vi "DebugView.vi"(10 "Compiled.Settings.ctl":T1, 11 "appended array":T8(array[cluster]) {"VS Refs" format="%.0x"}) -> ()   [LabVIEW 2019]
uses:
  <vilib>/NI VeriStand/Custom Device API/Custom Device Item Ref.ctl
  Shared/Compiled.Settings.ctl
  Shared/main_page_config.ctl
  Shared/object_managament_config.ctl
  Shared/interaction_parameter_configuration.ctl
  Shared/object_attribute_configuration.ctl
  Shared/object_status_info.ctl
  <vilib>/NI VeriStand/Custom Device API/Custom Device API.lvlib
  Shared/HLA Custom Device Shared.lvlib
panel:
  out "Compiled.Settings.ctl view":T1
  out "appended array view":T8(array[cluster]) {"VS Refs" format="%.0x"}
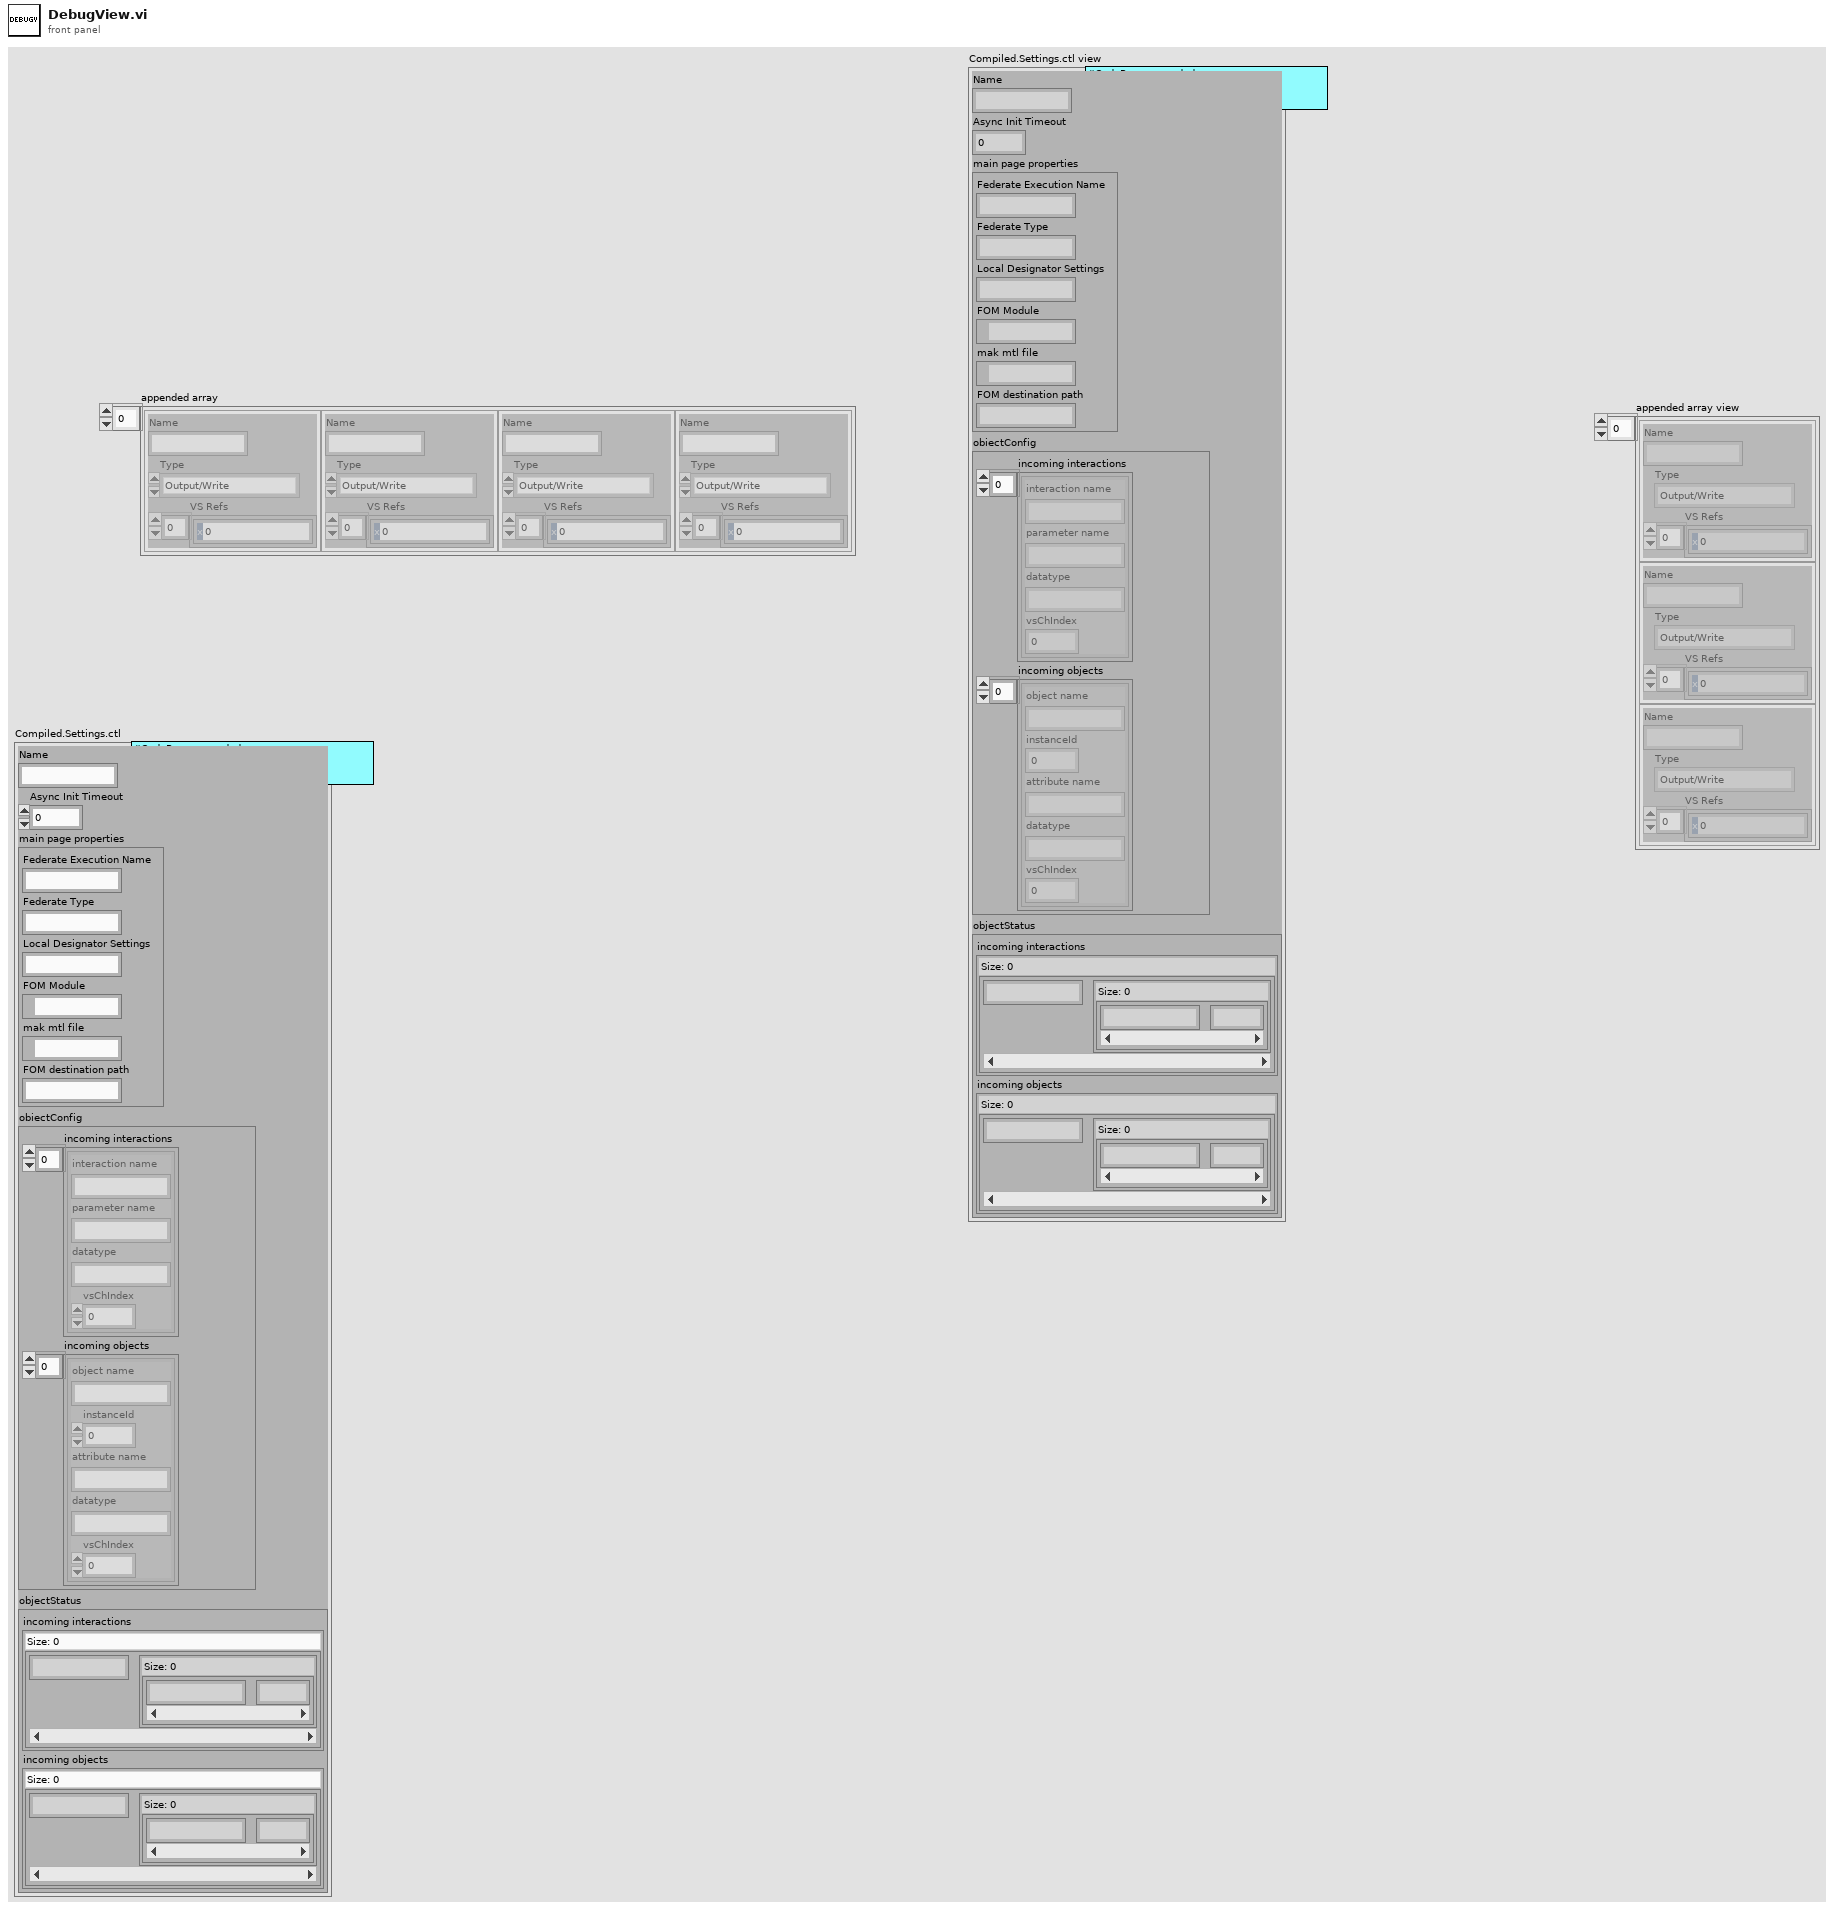
[diagram p1: front panel]
types:
  T1 = typedef "HLA Custom Device Shared.lvlib/Compiled.Settings.ctl" = cluster{"Name":string, "Async Init Timeout":u16, "main page properties":T2, "obiectConfig":T3, "objectStatus":T6}
  T2 = typedef "HLA Custom Device Shared.lvlib/main_page_config.ctl" = cluster{"Federate Execution Name":string, "Federate Type":string, "Local Designator Settings":string, "FOM Module":path, "mak mtl file":path, "FOM destination path":string}
  T3 = typedef "HLA Custom Device Shared.lvlib/object_managament_config.ctl" = cluster{"incoming interactions":T4[], "incoming objects":T5[]}
  T4 = typedef "HLA Custom Device Shared.lvlib/interaction_parameter_configuration.ctl" = cluster{"interaction name":string, "parameter name":string, "datatype":string, "vsChIndex":i32}
  T5 = typedef "HLA Custom Device Shared.lvlib/object_attribute_configuration.ctl" = cluster{"object name":string, "instanceId":i32, "attribute name":string, "datatype":string, "vsChIndex":i32}
  T6 = typedef "HLA Custom Device Shared.lvlib/object_status_info.ctl" = cluster{"incoming interactions":map{string, map{string, i32}}, "incoming objects":map{string, map{string, i32}}}
  T7 = typedef "Custom Device API.lvlib/Custom Device Item Ref.ctl" = u64
  T8 = cluster{"Name":string, "Type":enum16{"Output/Write", "Input/Read", "Input/ReadWrite"}, "VS Refs":T7[]}[]
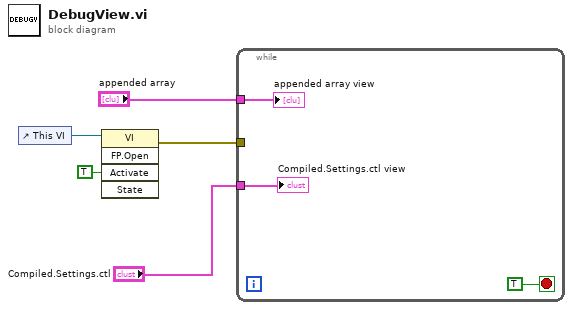
[diagram p0: block diagram]
diagram:
  n1 = control-ref of="This VI"() -> (w5:refnum<vi>)
  n2 = invoke class="VI" method="FP.Open"(reference=w5, "Activate"=TRUE ("Activate?")) -> (error out=w1:errorcluster)  [unwired: 3 in, 4 out]
  n3 = while {
    tunnel: "appended array" -> [w8]
    tunnel: "Compiled.Settings.ctl" -> [w7]
    tunnel: w1 -> [_]
    stop <- TRUE stop-if-true
    "appended array view" <- w8
    "Compiled.Settings.ctl view" <- w7
  }
